vi "Configure Analog Gen Log Sine Chirp.vi"(6 "Amplitude (0 Vrms)":dbl, 7 "FFT Source (0: csA0FFT)":i32(ring) items=["A0 FFT", "A0 FFT2Ch", "A1 FFT", "A1 FFT2Ch"], 8 "error in (no error)":errorcluster, 9 "Enable Waveform (T: Enable)":bool=TRUE, 10 "Channel (0: A)":i32(ring) items=["A", "B"], 11 "VISA resource name":refnum<visa-resource-name>) -> (0 "error out":errorcluster, 3 "VISA resource name out":refnum<visa-resource-name>)   [LabVIEW 2014, in "Stanford Research SR1.lvlib"]
doc: "Configures the attributes of the Analog Generator Log Sine Chirp."
uses:
  Stanford Research SR1.lvlib
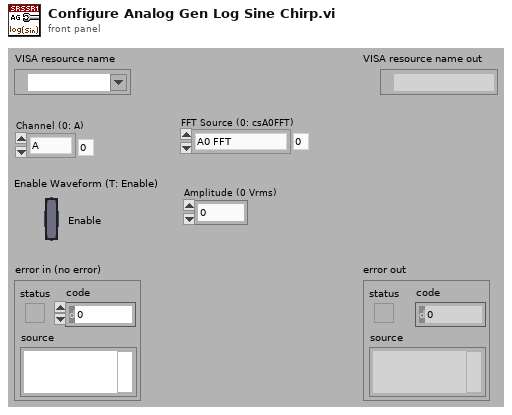
[diagram p1: front panel]
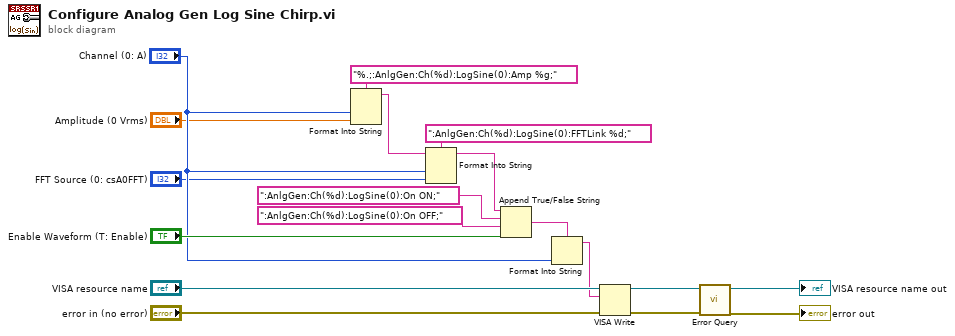
[diagram p0: block diagram]
diagram:
  n1 = Format Into String(format string="%.;:AnlgGen:Ch(%d):LogSine(0):Amp %g;", "Channel (0: A)", "Amplitude (0 Vrms)") -> (resulting string=w17:string)  [unwired: 2 in, 1 out]
  n2 = Format Into String(format string=":AnlgGen:Ch(%d):LogSine(0):FFTLink %d;", initial string=w17, "Channel (0: A)", "FFT Source (0: csA0FFT)") -> (resulting string=w15:string)  [unwired: 1 in, 1 out]
  n3 = Append True/False String(1:"Enable Waveform (T: Enable)", 2:":AnlgGen:Ch(%d):LogSine(0):On OFF;", 3:":AnlgGen:Ch(%d):LogSine(0):On ON;", 4:w15) -> (0:w5:string)
  n4 = Format Into String(format string=w5, "Channel (0: A)") -> (resulting string=w4:string)  [unwired: 2 in, 1 out]
  n5 = VISA Write(VISA resource name="VISA resource name", write buffer=w4, error in (no error)="error in (no error)") -> (VISA resource name out=w9:refnum<visa-resource-name>, error out=w8:errorcluster)  [unwired: 1 out]
  n6 = call "Error Query.vi"("error in (no error)"=w8, "VISA resource name"=w9) -> ("error out"=→"error out":errorcluster, "VISA resource name out"=→"VISA resource name out":refnum<visa-resource-name>)  [unwired: 6 in, 2 out]
